vi "Scripting_Server_driver.vi"(4 "error in (no error)":errorcluster, 6 "Action":enum16{"Launch", "Shutdown"}(ring)) -> (0 "error out":errorcluster)   [LabVIEW 2015]
doc: "Provides an interface to the Grating Translation Manager. See the actions below.\n\nLaunch - launch the manager thread supplying references to the controls that the thread will update.\n\nHome - Home the grating translation stage\n\nMove - Move the grating to the position supplied by Grating#\n\nShutdown - Shutdown the grating translation manager"
uses:
  Users/Sherman/Desktop/BETA_GSCS/Systems/SystemUtil/Command.ctl
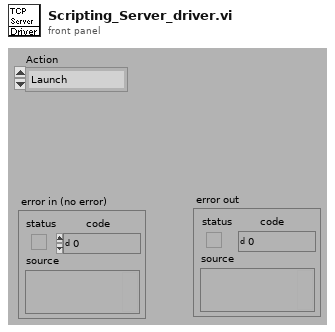
[diagram p1: front panel]
types:
  T1 = typedef "Command.ctl" = cluster{"Command":string, "Parameter":string}
  T2 = cluster{string, "type string":i16[], "data string":string}
  T3 = cluster{string, "type string":i16[], "data string":string}[]
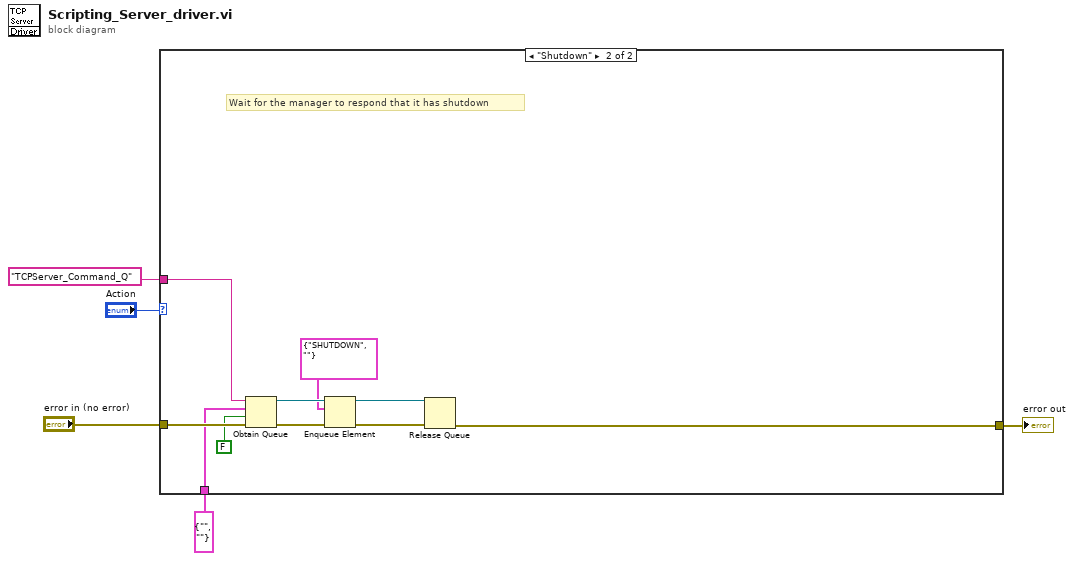
[diagram p0: block diagram]
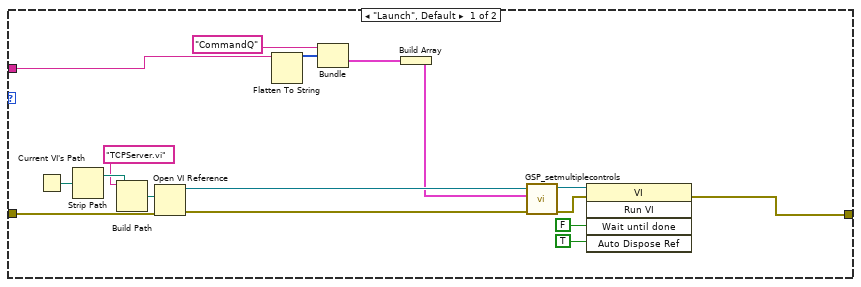
[diagram p2: hidden frame]
diagram:
  n1 = case shown="\"Shutdown\"" "Action" {
    tunnel: "error in (no error)" -> [w20 w33]
    tunnel: [w9 w24] -> w3
    tunnel: "TCPServer_Command_Q" -> [w10 w30]
    tunnel: T1 {"Command"="", "Parameter"=""} ("Command") -> [_ w28]
    frame "Launch", Default {
      n2 = Current VI's Path() -> (path=w14:path)
      n3 = Strip Path(path=w14) -> (stripped path=w12:path)  [unwired: 1 out]
      n4 = Build Path(base path=w12, name or relative path="TCPServer.vi" ("vi path")) -> (appended path=w13:path)
      n5 = Open VI Reference(vi path=w13, error in (no error)=w20) -> (vi reference=w8:refnum<vi>, error out=w19:errorcluster)  [unwired: 4 in]
      n6 = Flatten To String(anything=w10) -> (data string=w21:string, type string=w22:i16[])  [unwired: 3 in, 1 out]
      n7 = Bundle("CommandQ", "type string"=w22, "data string"=w21) -> (w7:T2)  [unwired: 1 in]
      n8 = Build Array(w7) -> (w6:T3)
      n9 = call "GSP_setmultiplecontrols.vi"("error in (no error)"=w19, "Control Infos"=w6, "reference"=w8) -> ("error out"=w17:errorcluster, "reference out"=w18:refnum<vi>)  [unwired: 3 in]
      n10 = invoke class="VI" method="Run VI"(reference=w18, error in=w17, "Wait until done"=FALSE, "Auto Dispose Ref"=TRUE) -> (error out=w9:errorcluster)  [unwired: 1 in, 4 out]
    }
    frame "Shutdown" {
      # "Wait for the manager to respond that it has shutdown"
      n11 = Obtain Queue(name (unnamed)=w30, element data type=w28, create if not found? (T)=FALSE, error in (no error)=w33) -> (queue out=w31:refnum<queue>, error out=w32:errorcluster)  [unwired: 1 in, 1 out]
      n12 = Enqueue Element(queue=w31, element=T1 {"Command"="SHUTDOWN", "Parameter"=""}, error in (no error)=w32) -> (queue out=w26:refnum<queue>, error out=w25:errorcluster)  [unwired: 1 in, 1 out]
      n13 = Release Queue(queue=w26, error in (no error)=w25) -> (error out=w24:errorcluster)  [unwired: 1 in, 2 out]
    }
  }
  "error out" <- w3
